vi "Format SQL INSERT.vi"(8 "error in":errorcluster, 9 "Time Stamp":timestamp, 10 "Data":variant, 11 "Path(s)":variant) -> (0 "error out":errorcluster, 2 "Formatted Insert":string)   [LabVIEW 2013, in "Data.PGSQL.lvclass"]
uses:
  Data.PGSQL.lvclass
  Typedefs/Errors--enum.ctl
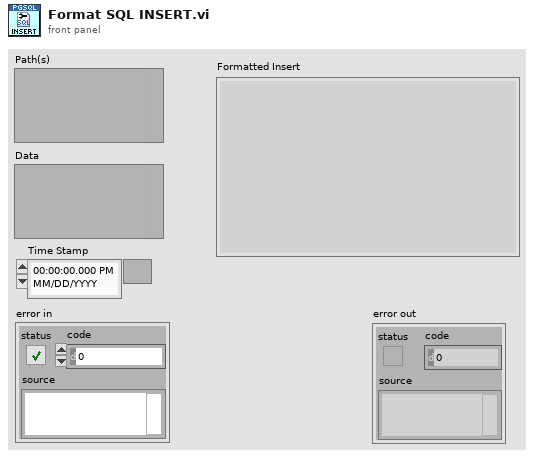
[diagram p1: front panel]
types:
  T1 = typedef "Data.PGSQL.lvclass/Errors--enum.ctl" = enum16{"0: None", "5005: Path Type Not Supported", "5006: Number of Variables", "5008: Cannot write two data points", "5030: Start and End Times Identical", "5031: Input is not wholly", "5033: Bad path or paths", "5040: Invalid Instrument Name", "5050: Column can only hold string", "5051 Column can only hold bool", "5052: Column can only hold double", "5053: Column can only hold int"}
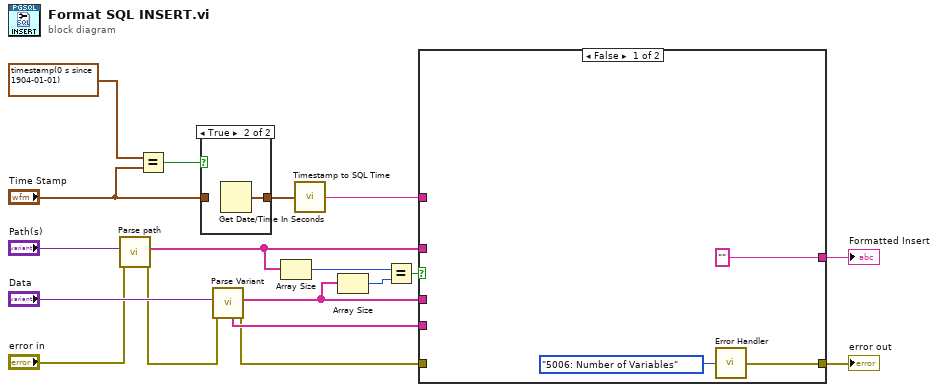
[diagram p0: block diagram]
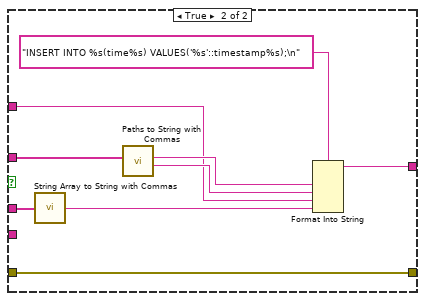
[diagram p2: hidden frame]
diagram:
  n1 = call "Parse path.vi"("error in"="error in", "Paths?"="Path(s)") -> ("error out"=w7:errorcluster, "Paths"=w1:string[])  [unwired: 8 in]
  n2 = Equal?(x=timestamp(0 s since 1904-01-01), y="Time Stamp") -> (x = y?=w17:bool)
  n3 = case shown="True" w17 {
    tunnel: [w19 w20] -> w6
    tunnel: "Time Stamp" -> [w19 _]
    frame False {
    }
    frame True {
      n4 = Get Date/Time In Seconds() -> (seconds since 1Jan1904=w20:timestamp)
    }
  }
  n5 = call "Parse Variant.vi"("error in"=w7, "variant"="Data") -> ("error out"=w2:errorcluster, "Strings"=w12:string[], "Types (strings)"=w4:string[])  [unwired: 5 in, 2 out]
  n6 = Array Size(array=w1) -> (size(s)=w15:i32)
  n7 = call "Timestamp to SQL Time.vi"("seconds since 1Jan1904"=w6) -> ("date/time string"=w5:string)
  n8 = Array Size(array=w12) -> (size(s)=w14:i32)
  n9 = Equal?(x=w15, y=w14) -> (x = y?=w13:bool)
  n10 = case shown="False" w13 {
    tunnel: w12 -> [_ w32]
    tunnel: w1 -> [_ w31]
    tunnel: [w22 w25] -> w11
    tunnel: w2 -> [_ w25]
    tunnel: w5 -> [_ w27]
    tunnel: w4 -> [_ _]
    tunnel: ["" w26] -> w9
    frame False {
      n11 = call "Error Handler.vi"("Error code"=Errors--enum."5006: Number of Variables") -> ("error out"=w22:errorcluster)
    }
    frame True {
      n12 = call "String Array to String with Commas.vi"("Array"=w32) -> ("String"=w28:string)
      n13 = call "Paths to String with Commas.vi"("Array"=w31) -> ("Columns"=w29:string, "Table"=w30:string)  [unwired: 9 in]
      n14 = Format Into String(format string="INSERT INTO %s(time%s) VALUES('%s'::timestamp%s);\n", w30, w29, w27, w28) -> (resulting string=w26:string)  [unwired: 2 in, 1 out]
    }
  }
  "error out" <- w11
  "Formatted Insert" <- w9
